vi "Write Registers.vi"(8 "error in (no error)":errorcluster, 9 "Data":u8[](array[numeric]), 10 "Registers":T1 items=["IODIRA"], 11 "MCP23017 in":refnum<class "MCP23017.lvclass">) -> (0 "error out":errorcluster, 3 "MCP23017 out":refnum<class "MCP23017.lvclass">)   [LabVIEW 2020, in "MCP23017.lvclass"]
uses:
  MCP23017.lvclass
  Registers.ctl
  MCP23017.lvclass/MCP23017.ctl
  I2C Bus Interface/I2C Bus.lvclass
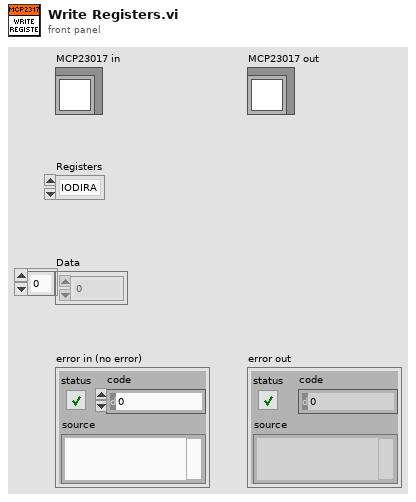
[diagram p1: front panel]
types:
  T1 = typedef "MCP23017.lvclass/Registers.ctl" = u16
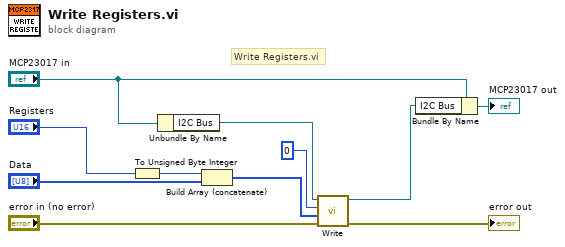
[diagram p0: block diagram]
diagram:
  # "Write Registers.vi"
  n1 = To Unsigned Byte Integer(number="Registers") -> (unsigned 8bit integer=w1:u8)
  n2 = Unbundle By Name("MCP23017 in") -> ("I2C Bus"=w5:refnum<class "I2C Bus.lvclass">)
  n3 = Build Array (concatenate)(w1, "Data") -> (w9:u8[])
  n4 = call-dynamic "Write.vi"("error in (no error)"="error in (no error)", "Data"=w9, "Address"=u8 0, "I2C Bus In"=w5) -> ("error out"=→"error out":errorcluster, "I2C Bus Out"=w8:refnum<class "I2C Bus.lvclass">)  [unwired: 6 in]
  n5 = Bundle By Name(cluster="MCP23017 in", "I2C Bus"=w8) -> (→"MCP23017 out":refnum<class "MCP23017.lvclass">)
